vi "Weather Station UI.vi"() -> ()   [LabVIEW 2012]
doc: "This is the main VI in the Weather Station project. It contains the user interface for a temperature warning system. Temperature is retrieved every half second; data is logged when a warning has occurred."
uses:
  Supporting Files/Weather Station States.ctl
  Supporting Files/Weather Data.ctl
  Instance           2 26Saved   Weather Station UI .vi
panel:
  out "Warning":string
  in  "Lower Limit":dbl=20.0
  in  "Upper Limit":dbl=30.0
  in  "Stop Button":bool
  out "Temperature History":dbl(graph)
  # "Temperature Ranges (C)"
  # "Freeze"
  # "Heat \nStroke"
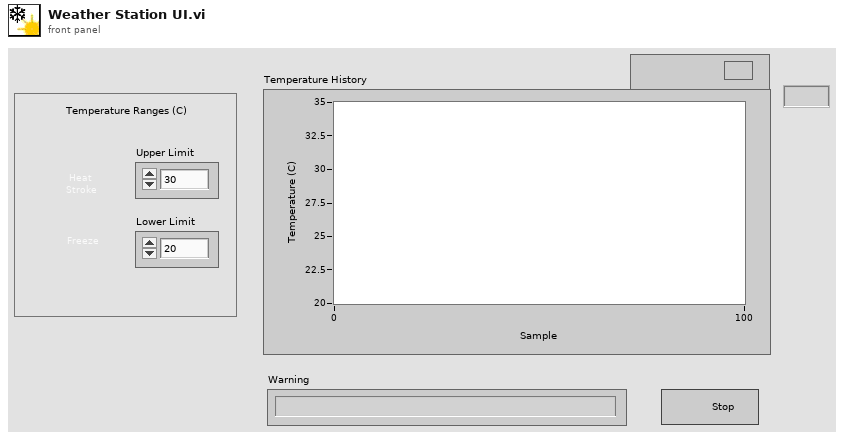
[diagram p1: front panel]
types:
  T1 = typedef "Weather Data.ctl" = cluster{"Current Temperature":dbl, "Max Temperature":dbl, "Min Temperature":dbl, "Temperature Warning?":bool, "Temperature Warning Text":string}
  T2 = typedef "Weather Station States.ctl" = enum16{"Acquisition", "Range Clock", "Analysis", "Data Log", "Time Check"}
  T3 = enum16{"open", "replace", "create", "open or create", "replace or create", "replace or create with confirmation"}
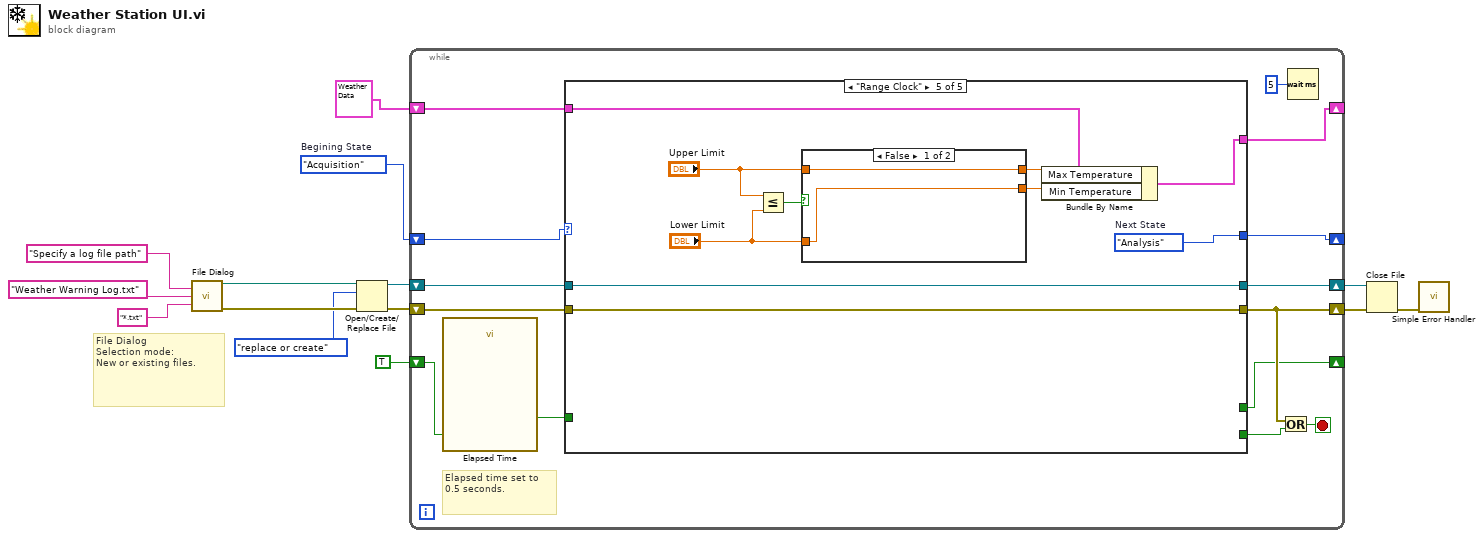
[diagram p0: block diagram]
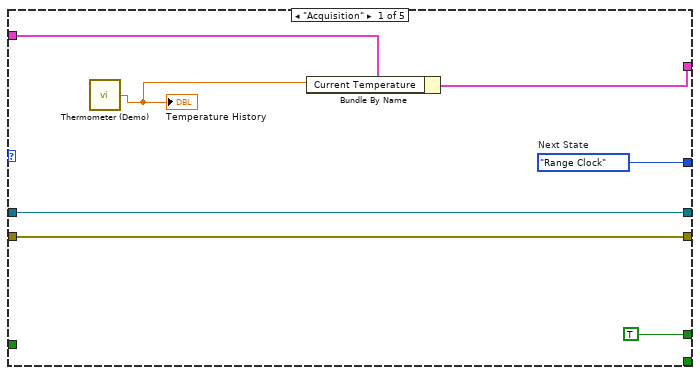
[diagram p2: hidden frame]
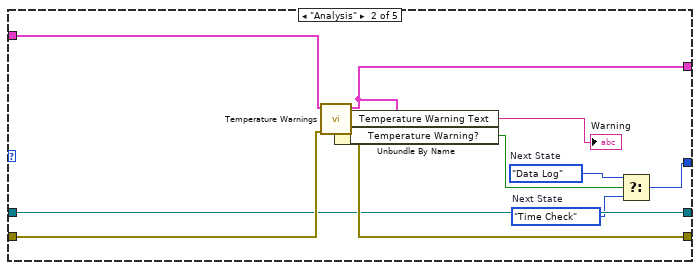
[diagram p3: hidden frame]
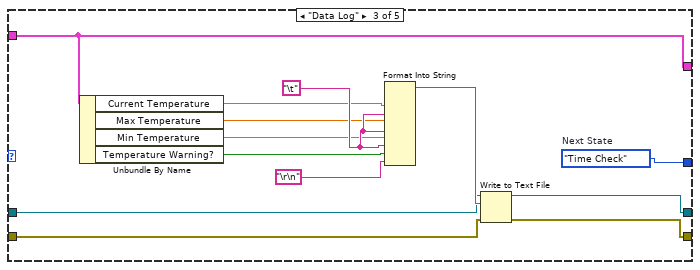
[diagram p4: hidden frame]
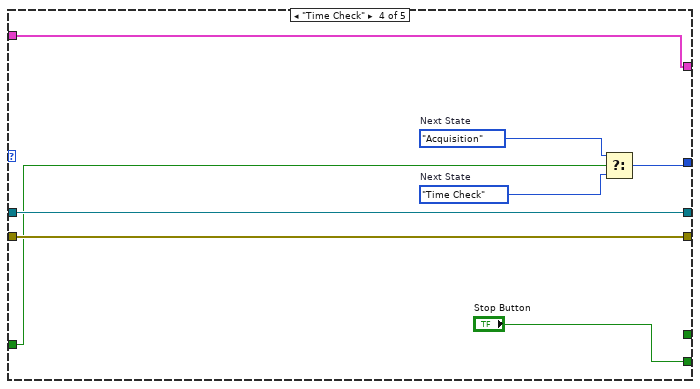
[diagram p5: hidden frame]
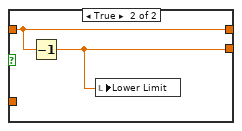
[diagram p6: hidden frame]
diagram:
  w2 = Weather_Station_States."Acquisition"  # Begining State
  # "File Dialog\nSelection mode:\nNew or existing files."
  n1 = call "File Dialog"("prompt"="Specify a log file path", "default name"="Weather Warning Log.txt", "pattern (all files)"="*.txt" ("pattern label")) -> ("selected path"=w8:path, "error out"=w5:errorcluster)  [unwired: 9 in, 2 out]
  n2 = Open/Create/Replace File(file path (use dialog)=w8, error in=w5, operation (0:open)=T3."replace or create") -> (refnum out=w10:refnum<file>, error out=w9:errorcluster)  [unwired: 3 in, 1 out]
  n3 = while {
    shift-right: [w21] -> w14
    shift-left: w9 -> [w28]
    shift-right: [w26] -> w13
    shift-left: w10 -> [w25]
    shift-right: [w16] -> _
    shift-left: TRUE ("stop") -> [w23]
    shift-right: [w17] -> _
    shift-left: w2 -> [w20]
    shift-right: [w18] -> _
    shift-left: T1 {"Current Temperature"=0.0, "Max Temperature"=0.0, "Min Temperature"=0.0, "Temperature Warning?"=FALSE, "Temperature Warning Text"="No Warning"} ("Weather Data In") -> [w19]
    stop <- w27 stop-if-true
    # "Elapsed time set to\n0.5 seconds."
    n4 = call "Elapsed Time"("Reset"=w23) -> ("Time has Elapsed"=w22:bool)  [unwired: 11 in, 7 out]
    n5 = case shown="\"Range Clock\"" w20 {
      tunnel: [w34 w44 w47 w65 w74] -> w21
      tunnel: w28 -> [w34 w45 w48 w65 w74]
      tunnel: [w35 w41 w50 w64 w75] -> w26
      tunnel: w25 -> [w35 w41 w49 w64 w75]
      tunnel: w22 -> [_ _ _ w62 _]
      tunnel: w19 -> [w32 w36 w58 w66 w68]
      tunnel: [w31 w43 w58 w66 w67] -> w18
      tunnel: [w30 w39 w46 w63 w76] -> w17
      tunnel: [TRUE _ _ _ _] -> w16
      tunnel: [_ _ _ "Stop Button" _] -> w15
      frame "Acquisition" {
        w30 = Weather_Station_States."Range Clock"  # Next State
        n6 = call "Thermometer (Demo).vi"() -> ("Temperature Value"=w33:dbl)  [unwired: 1 in]
        "Temperature History" <- w33
        n7 = Bundle By Name(cluster=w32, "Current Temperature"=w33) -> (w31:T1)
      }
      frame "Analysis" {
        w38 = Weather_Station_States."Time Check"  # Next State
        w37 = Weather_Station_States."Data Log"  # Next State
        n8 = call "Temperature Warnings.vi"("Error In"=w45, "Weather Data In"=w36) -> ("Error Out"=w44:errorcluster, "Weather Data Out"=w43:T1)  [unwired: 8 in]
        n9 = Unbundle By Name(w43) -> ("Temperature Warning Text"=→"Warning":string, "Temperature Warning?"=w40:bool)
        n10 = Select(t=w37, s=w40, f=w38) -> (s? t:f=w39:T2)
      }
      frame "Data Log" {
        w46 = Weather_Station_States."Time Check"  # Next State
        w55 = "\t"
        n11 = Unbundle By Name(w58) -> ("Current Temperature"=w54:dbl, "Max Temperature"=w53:dbl, "Min Temperature"=w52:dbl, "Temperature Warning?"=w56:bool)
        n12 = Format Into String(w54, w55, w53, w55, w52, w55, w56, "\r\n") -> (resulting string=w51:string)  [unwired: 3 in, 1 out]
        n13 = Write to Text File(file (use dialog)=w49, text=w51, error in=w48) -> (refnum out=w50:refnum<file>, error out=w47:errorcluster)  [unwired: 1 in, 1 out]
      }
      frame "Time Check" {
        w60 = Weather_Station_States."Time Check"  # Next State
        w61 = Weather_Station_States."Acquisition"  # Next State
        n14 = Select(t=w61, s=w62, f=w60) -> (s? t:f=w63:T2)
      }
      frame "Range Clock" {
        w76 = Weather_Station_States."Analysis"  # Next State
        n15 = Less Or Equal?(x="Upper Limit", y="Lower Limit") -> (x <= y?=w73:bool)
        n16 = case shown="False" w73 {
          tunnel: "Upper Limit" -> [w78 w80]
          tunnel: "Lower Limit" -> [w77 _]
          tunnel: [w78 w80] -> w70
          tunnel: [w77 w79] -> w69
          frame False {
          }
          frame True {
            n17 = Decrement(x=w80) -> (x-1=w79:dbl)
            n18 = local write "Lower Limit"(w79) -> ()
          }
        }
        n19 = Bundle By Name(cluster=w68, "Max Temperature"=w70, "Min Temperature"=w69) -> (w67:T1)
      }
    }
    n20 = Or(x=w21, y=w15) -> (x .or. y?=w27:bool)
    n21 = Wait (ms)(milliseconds to wait=u32 5 ("y")) -> ()  [unwired: 1 out]
  }
  n22 = Close File(refnum=w13, error in=w14) -> (error out=w12:errorcluster)  [unwired: 1 out]
  n23 = call <vilib>:"Simple Error Handler.vi"("error in (no error)"=w12) -> ()  [unwired: 4 in, 5 out]
